vi "Get Generation Regs.vi"(2 "gen":refnum<class "niUSRP Tx DSP v2 FPGA.lvclass">) -> (4 "dsp":T1 caption="misc")   [LabVIEW 2025, in "niUSRP Tx DSP v2 FPGA.lvclass"]
uses:
  niUSRP Tx DSP v2 FPGA.lvclass
  Typedefs/Tx DSP Shared Registers.ctl
  niUSRP Tx DSP v2 FPGA.lvclass/niUSRP Tx DSP v2 FPGA.ctl
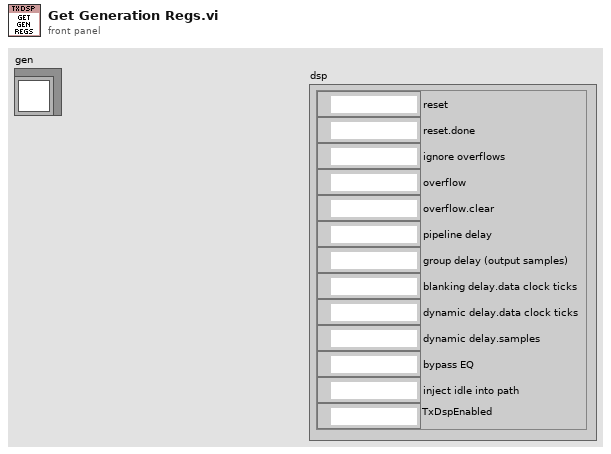
[diagram p1: front panel]
types:
  T1 = typedef "niUSRP Tx DSP v2 FPGA.lvclass/Tx DSP Shared Registers.ctl" = cluster{"reset":refnum<k21>, "reset.done":refnum<k21>, "ignore overflows":refnum<k21>, "overflow":refnum<k21>, "overflow.clear":refnum<k21>, "pipeline delay":refnum<k21>, "group delay (output samples)":refnum<k21>, "blanking delay.data clock ticks":refnum<k21>, "dynamic delay.data clock ticks":refnum<k21>, "dynamic delay.samples":refnum<k21>, "bypass EQ":refnum<k21>, "inject idle into path":refnum<k21>, "TxDspEnabled":refnum<k21>}
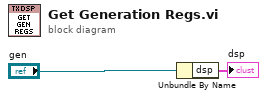
[diagram p0: block diagram]
diagram:
  n1 = Unbundle By Name("gen") -> ("dsp"=→"dsp":T1)
